vi "TestInitializeOneShotSubscription_RejectOldValue.vi"(8 "error in (no error)":errorcluster, 11 "TestCase in":refnum<class "TestSubscriptionPolicy.lvclass">) -> (0 "error out":errorcluster, 3 "TestCase out":refnum<class "TestSubscriptionPolicy.lvclass">)   [LabVIEW 2015, in "TestSubscriptionPolicy.lvclass"]
uses:
  TestSubscriptionPolicy.lvclass
  Framework/Mediator/SubscriptionPolicy/OneShotSubscription/OneShotSubscription.lvclass/OneShotSubscription.ctl
  Framework/Mediator/SubscriptionPolicy/OneShotSubscription/OneShotSubscription.lvclass
  Framework/Mediator/Transport/QueueTransport/QueueTransport.lvclass
  Framework/IMediator/ISubscriptionPolicy/ISubscriptionPolicy.lvclass
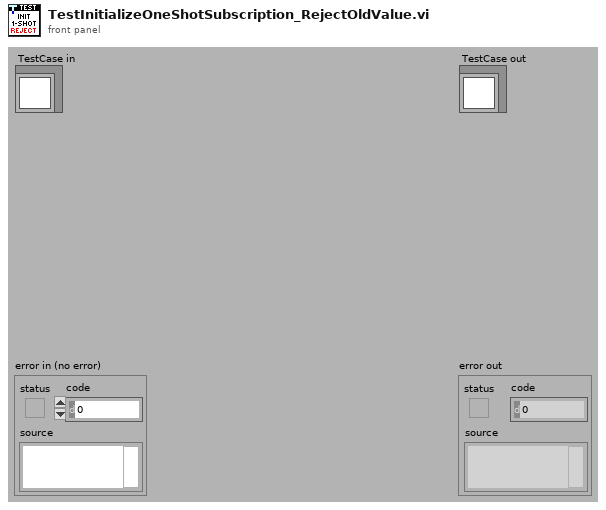
[diagram p1: front panel]
types:
  T1 = cluster{"Data":variant, "Publication Time":timestamp}
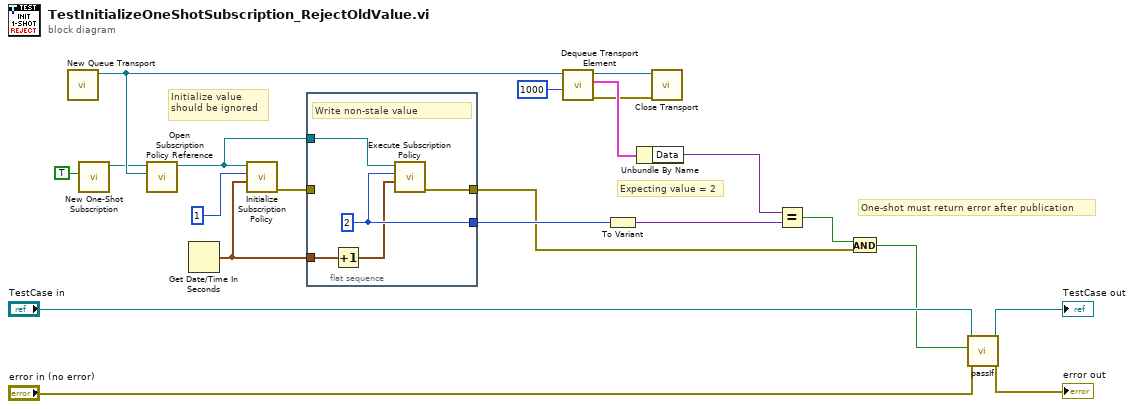
[diagram p0: block diagram]
diagram:
  # "Initialize value\nshould be ignored"
  # "One-shot must return error after publication"
  # "Expecting value = 2"
  n1 = call "New Queue Transport.vi"() -> ("QueueTransport Out"=w17:refnum<class "QueueTransport.lvclass">)  [unwired: 10 in, 1 out]
  n2 = call "New One-Shot Subscription.vi"("Ignore Past Updates? (F)"=TRUE) -> ("OneShotSubscription Out"=w12:refnum<class "OneShotSubscription.lvclass">)  [unwired: 10 in]
  n3 = call "Open Subscription Policy Reference.vi"("Transport"=w17, "SubscriptionPolicy"=w12) -> ("Subscription Policy"=w4:refnum<data-value>)  [unwired: 8 in, 1 out]
  n4 = Get Date/Time In Seconds() -> (seconds since 1Jan1904=w2:timestamp)
  n5 = call "Initialize Subscription Policy.vi"("Last Publish Time"=w2, "Last Topic Value"=1, "Subscription Policy"=w4) -> ("Error Out (Do Not Subscribe?)"=w1:errorcluster)  [unwired: 8 in]
  n6 = flat-sequence {
    tunnel: [w26] -> w9
    tunnel: [w25] -> w6
    tunnel: w4 -> [w24]
    tunnel: w2 -> [w23]
    tunnel: w1 -> [_]
    frame #0 {
      w26 = 2
      # "Write non-stale value"
      n7 = Increment(x=w23) -> (x+1=w22:timestamp)
      n8 = call "Execute Subscription Policy.vi"("Publish Time"=w22, "New Topic Value"=w26, "Subscription Policy"=w24) -> ("error out (Unsubscribe?)"=w25:errorcluster)  [unwired: 8 in]
    }
  }
  n9 = call "Dequeue Transport Element.vi"("Timeout In ms (-1)"=1000, "QueueTransport in"=w17) -> ("error out"=w13:errorcluster, "Element"=w15:T1, "QueueTransport out"=w14:refnum<class "QueueTransport.lvclass">)  [unwired: 6 in, 1 out]
  n10 = To Variant(anything=w9) -> (Variant=w8:variant)
  n11 = Unbundle By Name(w15) -> ("Data"=w10:variant)
  n12 = call-dynamic "Close Transport.vi"("error in (no error)"=w13, "QueueTransport in"=w14) -> ()  [unwired: 9 in, 1 out]
  n13 = Equal?(x=w10, y=w8) -> (x = y?=w7:bool)
  n14 = And(x=w7, y=w6) -> (x .and. y?=w5:bool)
  n15 = call-dynamic "passIf.vi"("error in (no error)"="error in (no error)", "pass"=w5, "TestCase in"="TestCase in") -> ("error out"=→"error out":errorcluster, "TestCase out"=→"TestCase out":refnum<class "TestSubscriptionPolicy.lvclass">)  [unwired: 7 in]
